vi "Read Data.vi"(1 "Channel Number":i32, 2 "GPIB Address":string, 3 "Number of Datapoints":i32) -> (0 "Data":i32[](array[numeric]))   [LabVIEW 2011]
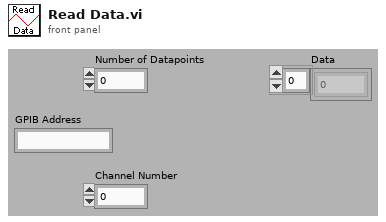
[diagram p1: front panel]
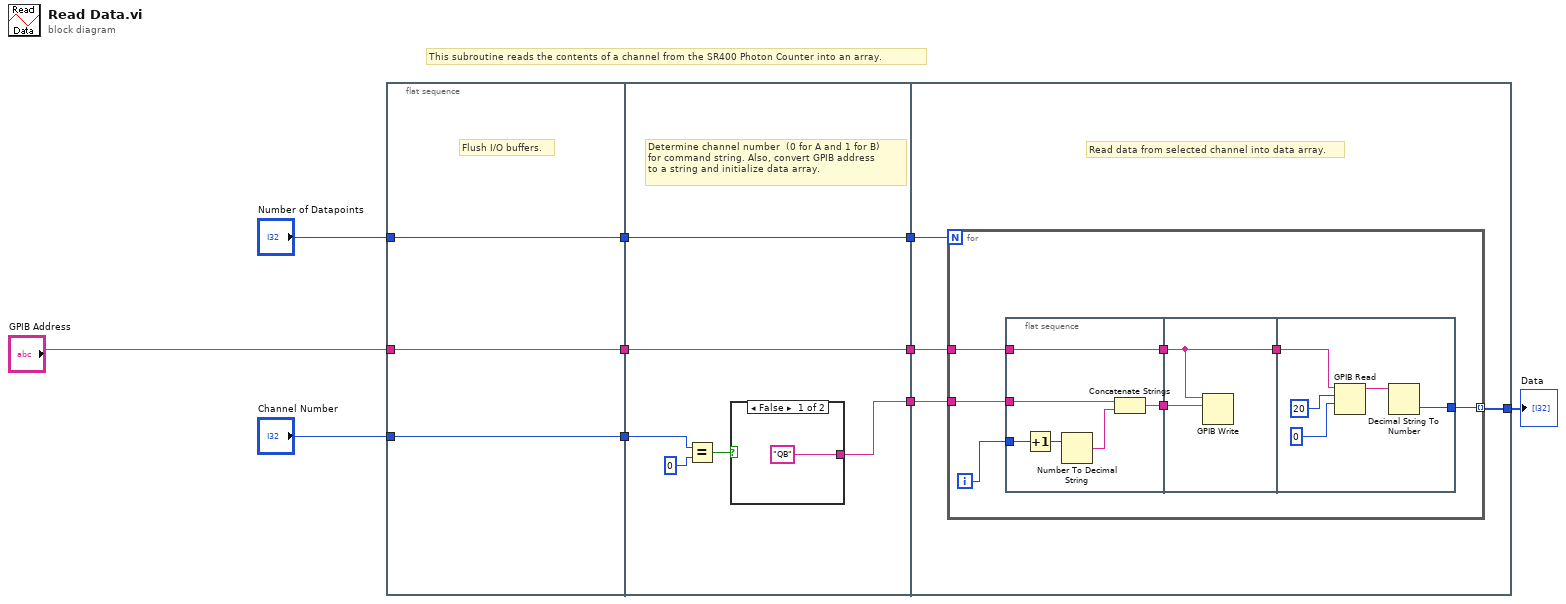
[diagram p0: block diagram]
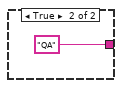
[diagram p2: hidden frame]
diagram:
  # "This subroutine reads the contents of a channel from the SR400 Photon Counter into an array."
  n1 = flat-sequence {
    tunnel: "GPIB Address" -> [w11]
    tunnel: "Number of Datapoints" -> [w12]
    tunnel: "Channel Number" -> [w13]
    tunnel: [w13] -> w3
    tunnel: [w12] -> w2
    tunnel: [w11] -> w1
    tunnel: [w16] -> w7
    tunnel: [w15] -> w6
    tunnel: [w14] -> w5
    tunnel: w3 -> [w17]
    tunnel: w2 -> [w14]
    tunnel: w1 -> [w15]
    tunnel: w7 -> [w25]
    tunnel: w6 -> [w24]
    tunnel: w5 -> [w23]
    tunnel: [w22] -> w4
    frame #0 {
      # "Flush I/O buffers."
    }
    frame #1 {
      # "Determine channel number  (0 for A and 1 for B) \nfor command string. Also, convert GPIB address\nto a string and initialize data array."
      n2 = Equal?(x=w17, y=0) -> (x = y?=w19:bool)
      n3 = case shown="False" w19 {
        tunnel: ["QB" "QA"] -> w16
        frame False {
        }
        frame True {
        }
      }
    }
    frame #2 {
      # "Read data from selected channel into data array."
      n4 = for {
        N: w23 -> [_]
        tunnel: w25 -> [w31]
        tunnel: w24 -> [w29]
        tunnel: [w27] -> w22 mode=indexing
        i -> [w32]
        n5 = flat-sequence {
          tunnel: w32 -> [w36]
          tunnel: w31 -> [w35]
          tunnel: [w34] -> w30
          tunnel: w29 -> [w33]
          tunnel: [w33] -> w28
          tunnel: w30 -> [w40]
          tunnel: w28 -> [w39]
          tunnel: [w39] -> w26
          tunnel: [w42] -> w27
          tunnel: w26 -> [w41]
          frame #0 {
            n6 = Increment(x=w36) -> (x+1=w37:i32)
            n7 = Number To Decimal String(number=w37) -> (decimal integer string=w38:string)  [unwired: 1 in]
            n8 = Concatenate Strings(w35, w38) -> (w34:string)
          }
          frame #1 {
            n9 = GPIB Write(0:w39, 1:w40) -> ()  [unwired: 3 in, 2 out]
          }
          frame #2 {
            n10 = GPIB Read(0:w41, 1:20, 2:0) -> (5:w45:string)  [unwired: 2 in, 2 out]
            n11 = Decimal String To Number(string=w45) -> (number=w42:i32)  [unwired: 2 in, 1 out]
          }
        }
      }
    }
  }
  "Data" <- w4
